vi "Extract BBM Slot Reference.vi"(10 "Slot":i32, 11 "Cluster in":refnum<vi>) -> (3 "Populated Reference":refnum<vi>)   [LabVIEW 2011]
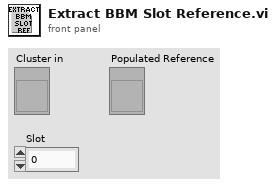
[diagram p1: front panel]
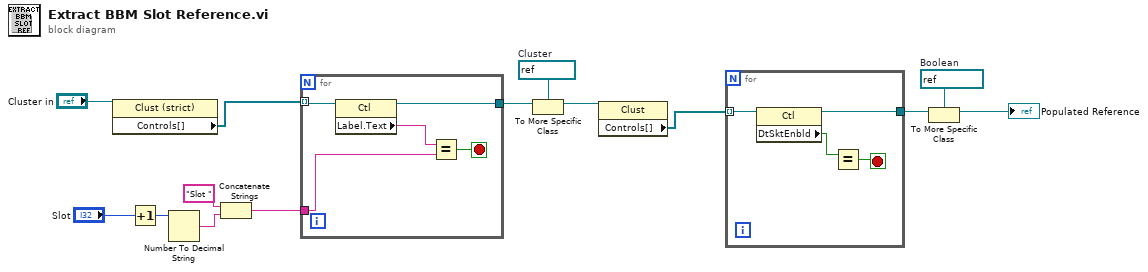
[diagram p0: block diagram]
diagram:
  w13 = refnum<vi> refnum  # Boolean
  w9 = refnum<vi> refnum  # Cluster
  n1 = property class="Clust (strict)"(reference="Cluster in") -> ("Controls[]"=w7:refnum<vi>[])  [unwired: 1 in, 2 out]
  n2 = Increment(x="Slot") -> (x+1=w3:i32)
  n3 = Number To Decimal String(number=w3) -> (decimal integer string=w4:string)  [unwired: 1 in]
  n4 = Concatenate Strings("Slot " ("string"), w4) -> (w6:string)
  n5 = for {
    tunnel: w6 -> [w18]
    tunnel: [w16] -> w8
    tunnel: w7 -> [w15] mode=indexing
    stop <- w17 stop-if-true
    n6 = property class="Ctl"(reference=w15) -> (reference out=w16:refnum<vi>, "Label.Text"=w19:string)  [unwired: 1 in, 1 out]
    n7 = Equal?(x=w19, y=w18) -> (x = y?=w17:bool)
  }
  n8 = To More Specific Class(target class=w9, reference=w8) -> (specific class reference=w10:refnum<vi>)  [unwired: 1 in, 1 out]
  n9 = property class="Clust"(reference=w10) -> ("Controls[]"=w11:refnum<vi>[])  [unwired: 1 in, 2 out]
  n10 = for {
    tunnel: w11 -> [w23] mode=indexing
    tunnel: [w20] -> w12
    stop <- w21 stop-if-true
    n11 = property class="Ctl"(reference=w23) -> (reference out=w20:refnum<vi>, "DtSktEnbld"=w22:bool)  [unwired: 1 in, 1 out]
    n12 = Equal?(x=w22) -> (x = y?=w21:bool)  [unwired: 1 in]
  }
  n13 = To More Specific Class(target class=w13, reference=w12) -> (specific class reference=→"Populated Reference":refnum<vi>)  [unwired: 1 in, 1 out]
